vi "COM UUT Board.vi"(8 "error in (no error)":errorcluster, 10 "VI reference (current VI)":refnum<vi>, 11 "VISA resource name 2":refnum<visa-resource-name>) -> (0 "error out":errorcluster, 2 ".not. x?":bool, 3 "VISA resource name out":refnum<visa-resource-name>)   [LabVIEW 2017]
uses:
  <vilib>/Instr/_visa.llb/VISA Configure Serial Port (Instr).vi
panel:
  in  "Blank Button":bool
  in  "VISA resource name":refnum<visa-resource-name>
  # "Please choose the UUT COM Port"
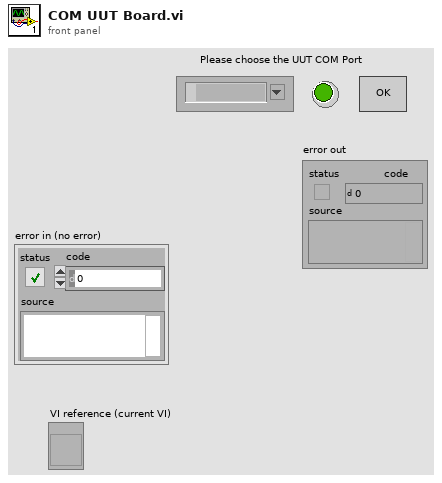
[diagram p1: front panel]
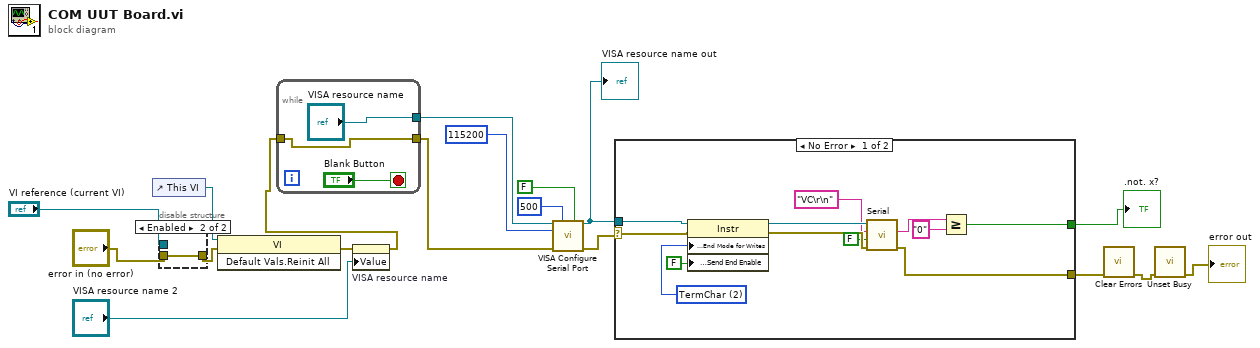
[diagram p0: block diagram]
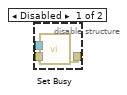
[diagram p2: hidden frame]
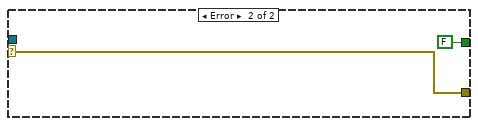
[diagram p3: hidden frame]
diagram:
  n1 = control-ref of="This VI"() -> (w18:refnum<vi>)
  n2 = disable-structure shown="Enabled" {
    disable-tunnel: "VI reference (current VI)" -> [w21 _]
    disable-tunnel: "error in (no error)" -> [w20 w22]
    disable-tunnel: [w19 w22] -> w3
    frame Disabled {
      n3 = call <vilib>:"Set Busy.vi"("error in (no error)"=w20, "VI reference (current VI)"=w21) -> ("error out"=w19:errorcluster)  [unwired: 8 in, 1 out]
    }
    frame Enabled {
    }
  }
  n4 = invoke class="VI" method="Default Vals.Reinit All"(reference=w18, error in=w3) -> (error out=w17:errorcluster)  [unwired: 1 in, 2 out]
  n5 = property on="VISA resource name" class="VISAName"(error in=w17, "Value"="VISA resource name 2") -> (error out=w2:errorcluster)  [unwired: 1 in, 1 out]
  n6 = while {
    tunnel: ["VISA resource name"] -> w15
    tunnel: w2 -> [w23]
    tunnel: [w23] -> w1
    stop <- "Blank Button" stop-if-true
  }
  n7 = call-poly "VISA Configure Serial Port"("VISA resource name"=w15, "timeout (10sec)"=u32 500, "Enable Termination\nChar (T)"=FALSE ("Enable Termination\nChar (T)"), "baud rate (9600)"=u32 115200 ("baud rate"), "error in (no error)"=w1) -> ("VISA resource name out"=w11:refnum<visa-resource-name>, "error out"=w6:errorcluster)  [unwired: 9 in]
  "VISA resource name out" <- w11
  n8 = case shown="No Error" w6 {
    selector: w6 -> [w26 w38]
    tunnel: w11 -> [w29 _]
    tunnel: [w28 w38] -> w10
    tunnel: [w27 FALSE] -> w7
    frame No Error {
      w36 = u16 2 items=["None", "LastBit", "TermChar", "Break"] ("Serial Settings:Serial End Mode for Writes")
      n9 = property class="Instr"(reference=w29, error in=w26, "Serial Settings:End Mode for Writes"=w36, "Message Based Settings:Send End Enable"=FALSE) -> (reference out=w34:refnum<visa-resource-name>, error out=w35:errorcluster)
      n10 = call "Serial.vi"("error in (no error)"=w35, "Clear Log"=FALSE, "write buffer"="VC\r\n", "VISA resource name"=w34) -> ("error out"=w28:errorcluster, "read buffer"=w33:string)  [unwired: 6 in]
      n11 = Greater Or Equal?(x=w33, y="0") -> (x >= y?=w27:bool)
    }
    frame Error {
    }
  }
  ".not. x?" <- w7
  n12 = call <vilib>:"Clear Errors.vi"("error in (no error)"=w10) -> ("error out"=w9:errorcluster)  [unwired: 5 in, 1 out]
  n13 = call <vilib>:"Unset Busy.vi"("error in (no error)"=w9) -> ("error out"=→"error out":errorcluster)  [unwired: 10 in]
